vi "field emission sensor_65.vi"() -> ()   [LabVIEW 2014]
uses:
  Keithley 24XX/Public/Data/Read (Single Point).vi
  Keithley 24XX/Keithley 24XX.lvlib
  <userlib>/Nanonis Prog Interface V5/Nanonis Prog Interface.lvlib
panel:
  out "x+y":sgl
  in  "p ramp":dbl=10500.0
  out "amplitude":sgl(graph)
  in  "delay  coarse step":u32
  in  "Amplitude (V) (NaN=no change)":sgl=nan
  in  "Frequency (Hz) (NaN=no change)":sgl=nan format="%#_6p"
  in  "p Amplitude":dbl=2e-08 format="%#_6p"
  in  "amplitude max":sgl=1e-10 format="%#_6p"
  in  "Signal index (0-79)":i8=49
  out "amplitude":sgl=7.943678e-12 format="%#_6p"
  in  "dz":dbl=1e-09 format="%#_6p"
  in  "ramp delay (s)":dbl=10500.0
  out "ramp trigger":bool
  out "millisecond timer value":u32=183946603
  in  "Clear plots":bool
  out "z":dbl(graph)=1.0959994182086754e-07
  in  "Ramp":bool=TRUE
  in  "steps":sgl=5e-09 format="%#_6p"
  in  "Ramp to":sgl=2.45e-07 format="%#_6p"
  in  "I":sgl=5e-05 format="%#_6p"
  in  "PID":bool
  in  "p":sgl=0.005 format="%#_6p"
  in  "setpoint":sgl=2.5000006e-07 format="%#_3p"
  in  "max Current":sgl=1e-06 format="%#_6p"
  in  "setpoint approach":sgl=3e-08 format="%#_6p"
  in  "auto approach":bool
  in  "Number of steps":u16=1
  in  "withdraw tip":bool
  in  "coarse step":bool
  in  "Direction":enum16{"X +", "X -", "Y +", "Y -", "Z +", "Z -"}(ring)=enum."Z +"
  in  "Machine name (local machine IP)":string="localhost"
  in  "Z position [m]":dbl=1.0959994182086754e-07 max=1.096e-07 step=1.0 format="%_6p"
  out "current [A]":sgl=2.086008e-11 format="%#_6p"
  in  "time divider":dbl=60.0
  out "time elapsed":dbl=58.44645961125692
  in  "milliseconds to wait":u32=100
  in  "VISA resource name":refnum<visa-resource-name>="GPIB0::21::INSTR"
  in  "stop":bool
  in  "current multiplier":sgl=1.0
  out "Current":sgl(graph)=2.086008e-11
  # "STOP the VI during an Nanonis Auto Approach"
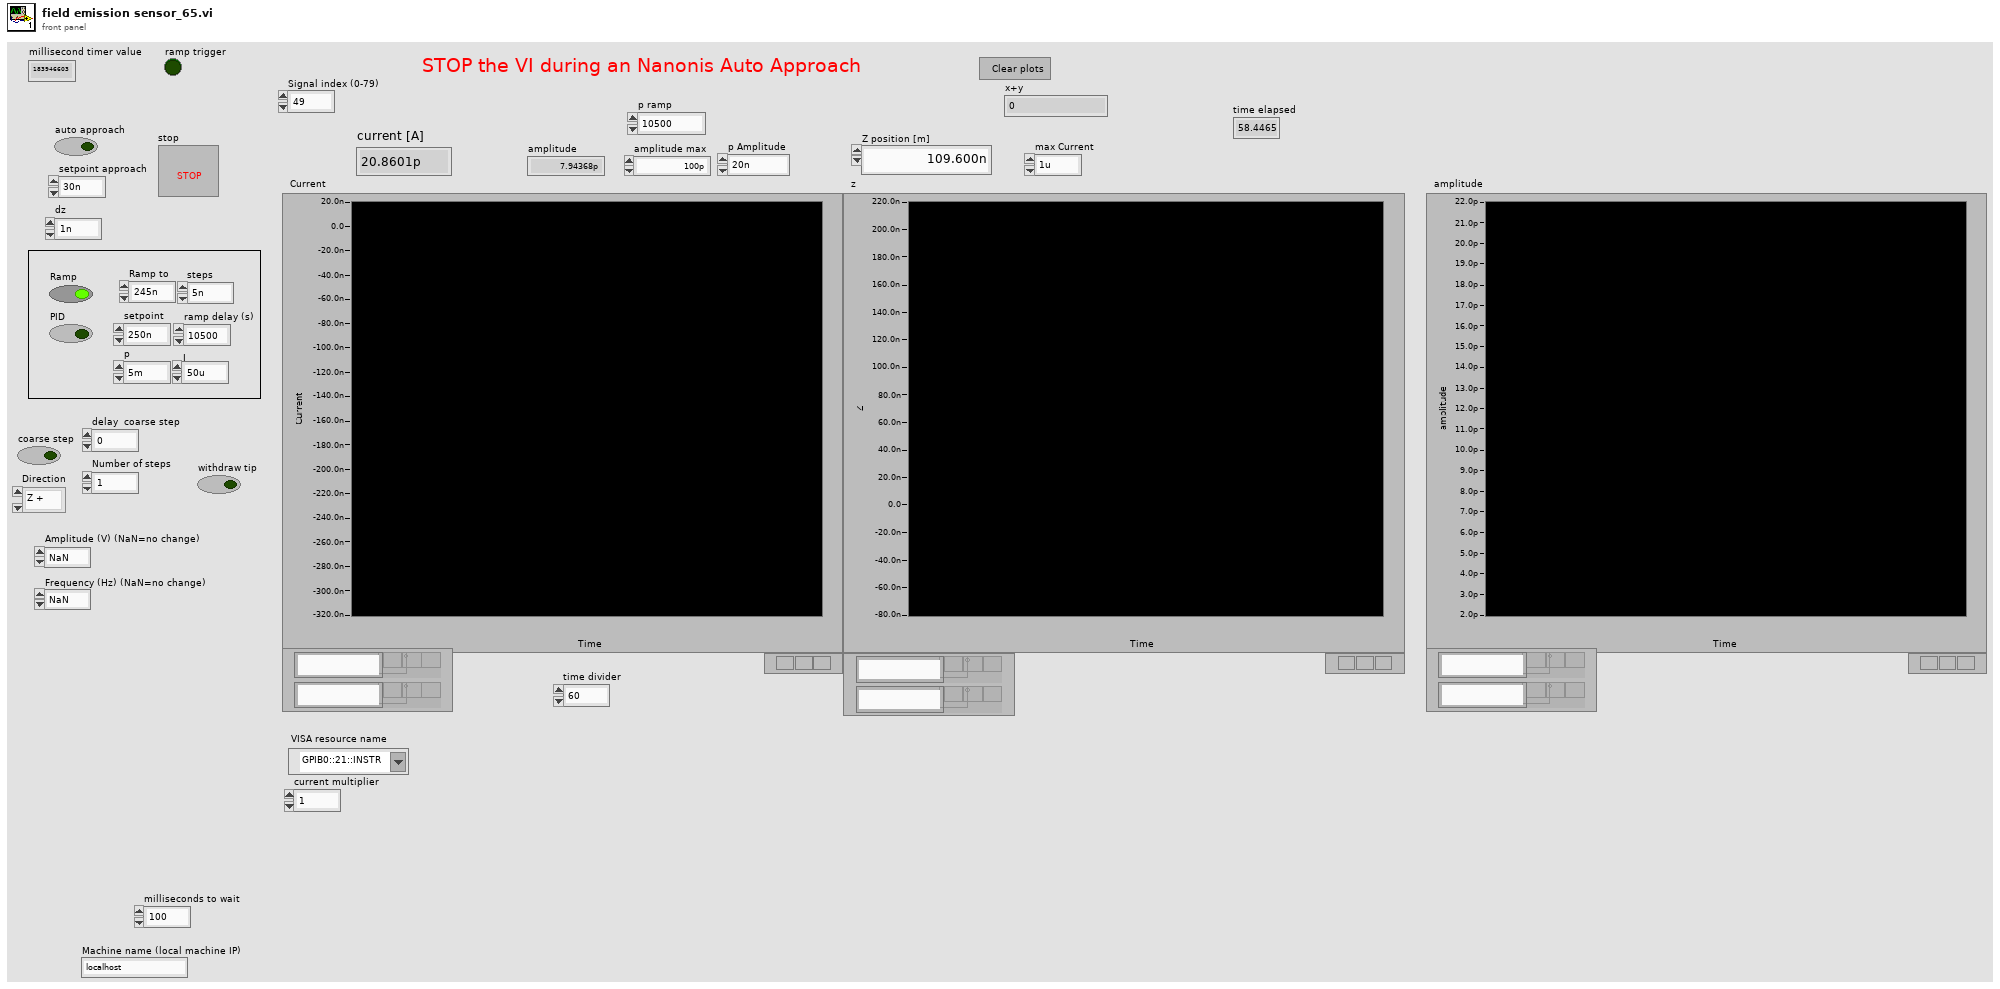
[diagram p1: front panel]
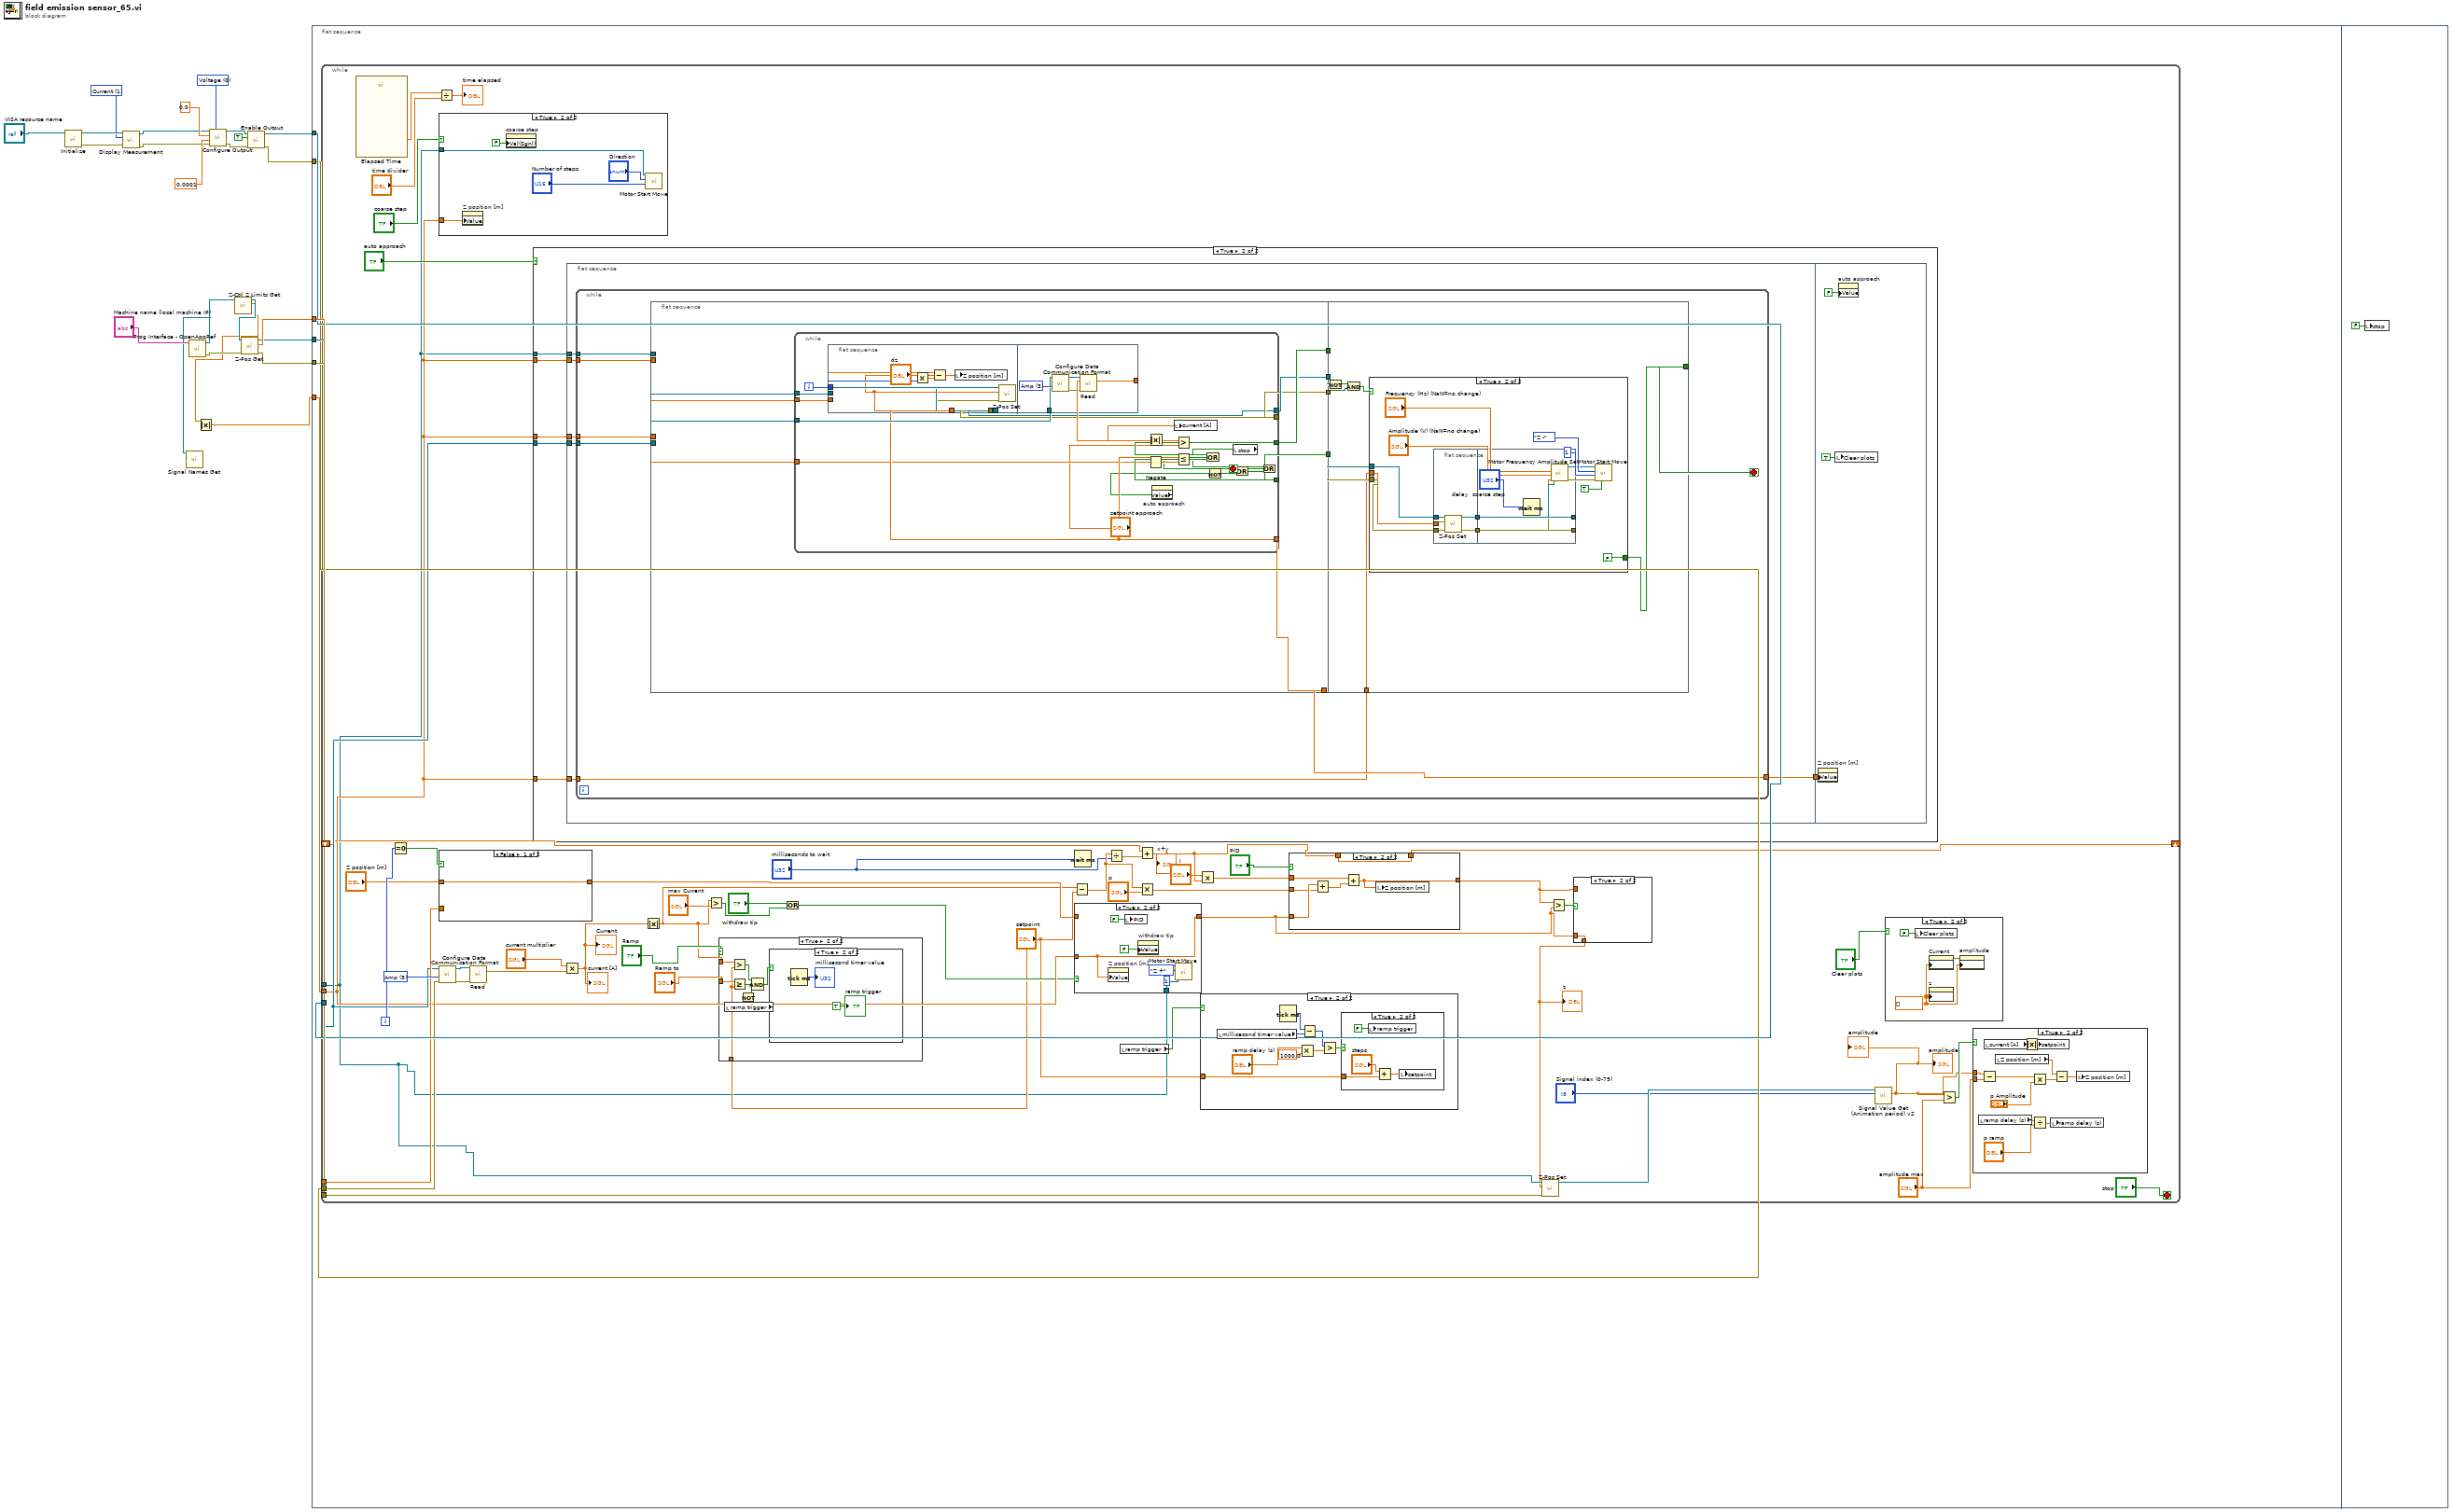
[diagram p0: block diagram]
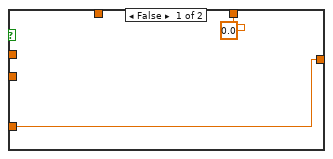
[diagram p9: hidden frame]
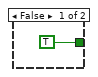
[diagram p11: hidden frame]
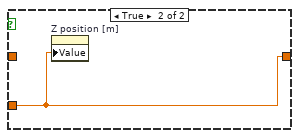
[diagram p14: hidden frame]
diagram:
  w5 = u16 1 items=["Voltage", "Current", "Resistance"] ("Displayed Measurement (0: Voltage)")
  w17 = u16 0 items=["Voltage", "Current"] ("Source Mode  (0: Voltage)")
  n1 = call "Initialize.vi"("VISA resource name"="VISA resource name") -> ("error out"=w7:errorcluster, "VISA resource name out"=w9:refnum<visa-resource-name>)  [unwired: 9 in]
  n2 = call "Display Measurement.vi"("error in (no error)"=w7, "Displayed Measurement (0: Voltage)"=w5, "VISA resource name"=w9) -> ("error out"=w6:errorcluster, "VISA resource name out"=w8:refnum<visa-resource-name>)  [unwired: 7 in]
  n3 = call <userlib>:"Prog Interface - OpenAppRef.vi"("Machine name (local machine IP)"="Machine name (local machine IP)") -> ("Error out"=w22:errorcluster, "Application reference"=w1:refnum<vi>)  [unwired: 5 in]
  n4 = call <userlib>:"Signal Names Get.vi"("Application ref in"=w1) -> ()  [unwired: 6 in, 3 out]
  n5 = call "Configure Output.vi"("Source Mode  (0: Voltage)"=w17, "error in (no error)"=w6, "Compliance  Level (0.1)"=0.0001, "Output Level (0)"=0.0, "VISA resource name"=w8) -> ("error out"=w13:errorcluster, "VISA resource name out"=w14:refnum<visa-resource-name>)  [unwired: 5 in]
  n6 = call <userlib>:"Z-Ctrl Z Limits Get.vi"("Application ref in"=w1) -> ("Z high limit"=w2:sgl, "Application ref out"=w3:refnum<vi>)  [unwired: 7 in, 2 out]
  n7 = Absolute Value(x=w2) -> (abs(x)=w4:sgl)
  n8 = call <userlib>:"Z-Pos Get.vi"("error in (no error)"=w22, "Application ref in"=w3) -> ("error out"=w21:errorcluster, "Z position (m)"=w20:sgl, "Application ref out"=w19:refnum<vi>)  [unwired: 7 in]
  n9 = call "Enable Output.vi"("error in (no error)"=w13, "Enable Output (T: Enable)"=TRUE, "VISA resource name"=w14) -> ("error out"=w10:errorcluster, "VISA resource name out"=w11:refnum<visa-resource-name>)  [unwired: 7 in]
  n10 = flat-sequence {
    tunnel: w21 -> [w29]
    tunnel: w20 -> [w28]
    tunnel: w19 -> [w27]
    tunnel: w11 -> [w26]
    tunnel: w10 -> [w25]
    tunnel: w4 -> [w24]
    frame #0 {
      n11 = while {
        tunnel: w27 -> [w34]
        tunnel: w29 -> [w73]
        tunnel: w28 -> [w72]
        tunnel: w26 -> [w64]
        tunnel: w25 -> [w63]
        tunnel: w24 -> [w61]
        shift-right: [w46] -> _
        shift-left: _ -> [w53]
        i -> [w71]
        stop <- "stop" stop-if-true
        w77 = u16 3 items=["All", "Volt and Amp", "Volt", "Amp"] ("Data Selection (0: All)")
        n12 = call "Elapsed Time"() -> ("Elapsed Time (s)"=w74:dbl)  [unwired: 12 in, 7 out]
        n13 = Equal To 0?(x=w71) -> (x = 0?=w70:bool)
        n14 = Divide(x=w74, y="time divider") -> (x/y=→"time elapsed":dbl)
        n15 = case shown="True" "coarse step" {
          tunnel: w34 -> [_ w240]
          tunnel: w61 -> [_ w236]
          frame False {
          }
          frame True {
            n16 = property on="Z position [m]" class="DigNum (strict)"("Value"=w236) -> ()  [unwired: 2 in, 2 out]
            n17 = property on="coarse step" class="Bool (strict)"("Val(Sgnl)"=FALSE ("Value (Signaling)")) -> ()  [unwired: 2 in, 2 out]
            n18 = call <userlib>:"Motor Start Move.vi"("Number of steps"="Number of steps", "Direction"="Direction", "Application ref in"=w240) -> ()  [unwired: 6 in, 2 out]
          }
        }
        n19 = case shown="False" w70 {
          tunnel: [w241 w242] -> w67
          tunnel: w72 -> [_ w242]
          tunnel: "Z position [m]" -> [w241 _]
          frame False {
          }
          frame True {
            n20 = property on="Z position [m]" class="DigNum (strict)"("Value"=w242) -> ()  [unwired: 2 in, 2 out]
          }
        }
        n21 = call "Configure Data Communication Format.vi"("error in (no error)"=w63, "Data Selection (0: All)"=w77, "VISA resource name"=w64) -> ("error out"=w78:errorcluster, "VISA resource name out"=w79:refnum<visa-resource-name>)  [unwired: 7 in]
        n22 = call-poly "Read.vi"("VISA resource name"=w79, "error in (no error)"=w78) -> ("Current"=w81:sgl)  [unwired: 7 in, 6 out]
        n23 = case shown="True" "auto approach" {
          tunnel: w64 -> [_ w134]
          tunnel: w34 -> [_ w133]
          tunnel: w61 -> [_ w131]
          tunnel: w61 -> [_ w130]
          tunnel: w61 -> [_ w129]
          frame False {
          }
          frame True {
            n24 = flat-sequence {
              tunnel: w134 -> [w140]
              tunnel: w133 -> [w139]
              tunnel: [w138] -> w132
              tunnel: w131 -> [w137]
              tunnel: w130 -> [w136]
              tunnel: w129 -> [w135]
              tunnel: w132 -> [w227]
              frame #0 {
                n25 = while {
                  tunnel: w140 -> [w151]
                  tunnel: w139 -> [w150]
                  tunnel: [w144] -> w138
                  tunnel: w137 -> [w143]
                  tunnel: w136 -> [w142]
                  tunnel: w135 -> [w141]
                  stop <- w145 stop-if-true
                  n26 = flat-sequence {
                    tunnel: w151 -> [w160]
                    tunnel: w150 -> [w159]
                    tunnel: [w158] -> w149
                    tunnel: [w157] -> w148
                    tunnel: [w156] -> w147
                    tunnel: [w155] -> w146
                    tunnel: [w154] -> w144
                    tunnel: w143 -> [w153]
                    tunnel: w141 -> [w152]
                    tunnel: w149 -> [w201]
                    tunnel: w148 -> [w199]
                    tunnel: w147 -> [w197]
                    tunnel: w146 -> [w196]
                    tunnel: [w195] -> w145
                    tunnel: w142 -> [w194]
                    frame #0 {
                      n27 = while {
                        tunnel: w160 -> [w179]
                        tunnel: w159 -> [w177]
                        tunnel: [w176] -> w158
                        tunnel: [w175] -> w157
                        tunnel: [w174] -> w156
                        tunnel: [w173] -> w155
                        tunnel: [w172] -> w154
                        tunnel: w153 -> [w171]
                        tunnel: w152 -> [w169]
                        i -> [w180]
                        stop <- w164 stop-if-true
                        n28 = flat-sequence {
                          tunnel: w180 -> [w188]
                          tunnel: w177 -> [w187]
                          tunnel: [w182] -> w172
                          tunnel: [w186] -> w174
                          tunnel: [w185] -> w173
                          tunnel: w171 -> [w184]
                          tunnel: w179 -> [w190]
                          tunnel: [w189] -> w178
                          frame #0 {
                            n29 = Multiply(x="dz", y=w188) -> (x*y=w183:dbl)
                            n30 = Subtract(x=w184, y=w183) -> (x-y=w182:dbl)
                            n31 = local write "Z position [m]"(w182) -> ()
                            n32 = call <userlib>:"Z-Pos Set.vi"("Z position (m)"=w182, "Application ref in"=w187) -> ("error out"=w185:errorcluster, "Application ref out"=w186:refnum<vi>)  [unwired: 8 in]
                          }
                          frame #1 {
                            w191 = u16 3 items=["All", "Volt and Amp", "Volt", "Amp"] ("Data Selection (0: All)")
                            n33 = call "Configure Data Communication Format.vi"("Data Selection (0: All)"=w191, "VISA resource name"=w190) -> ("error out"=w192:errorcluster, "VISA resource name out"=w193:refnum<visa-resource-name>)  [unwired: 8 in]
                            n34 = call-poly "Read.vi"("VISA resource name"=w193, "error in (no error)"=w192) -> ("Current"=w189:sgl)  [unwired: 7 in, 6 out]
                          }
                        }
                        n35 = Negate(x=w169) -> (-x=w170:sgl)
                        n36 = Absolute Value(x=w178) -> (abs(x)=w161:sgl)
                        n37 = property on="auto approach" class="Bool (strict)"() -> ("Value"=w167:bool)  [unwired: 2 in, 2 out]
                        n38 = local write "current [A]"(w161) -> ()
                        n39 = Greater?(x=w161, y="setpoint approach") -> (0:w176:bool)
                        n40 = Less Or Equal?(x=w172, y=w170) -> (x <= y?=w175:bool)
                        n41 = Or(x=w176, y=w175) -> (x .or. y?=w168:bool)
                        n42 = Not(x=w167) -> (.not. x?=w166:bool)
                        n43 = local read "stop"() -> (w163:bool)
                        n44 = Or(x=w168, y=w166) -> (x .or. y?=w165:bool)
                        n45 = Or(x=w163, y=w165) -> (x .or. y?=w164:bool)
                      }
                    }
                    frame #1 {
                      n46 = Not(x=w201) -> (.not. x?=w200:bool)
                      n47 = And(x=w200, y=w199) -> (x .and. y?=w198:bool)
                      n48 = case shown="True" w198 {
                        tunnel: w197 -> [_ w217]
                        tunnel: w196 -> [_ w216]
                        tunnel: [TRUE FALSE] -> w195
                        tunnel: w194 -> [_ w212]
                        frame False {
                        }
                        frame True {
                          n49 = flat-sequence {
                            tunnel: w217 -> [w222]
                            tunnel: w216 -> [w221]
                            tunnel: w212 -> [w220]
                            tunnel: [w219] -> w204
                            tunnel: [w218] -> w203
                            tunnel: [w224] -> w208
                            tunnel: [w225] -> w209
                            tunnel: w204 -> [w225]
                            tunnel: w203 -> [w224]
                            frame #0 {
                              n50 = call <userlib>:"Z-Pos Set.vi"("error in (no error)"=w221, "Z position (m)"=w220, "Application ref in"=w222) -> ("error out"=w218:errorcluster, "Application ref out"=w219:refnum<vi>)  [unwired: 7 in]
                            }
                            frame #1 {
                              n51 = Wait (ms)(milliseconds to wait="delay  coarse step") -> ()  [unwired: 1 out]
                            }
                          }
                          n52 = call <userlib>:"Motor Frequency Amplitude Set.vi"("Error in (no error)"=w208, "Amplitude (V) (NaN=no change)"="Amplitude (V) (NaN=no change)", "Frequency (Hz) (NaN=no change)"="Frequency (Hz) (NaN=no change)", "Application ref in"=w209) -> ("Error out"=w207:errorcluster, "Application ref out"=w210:refnum<vi>)  [unwired: 6 in]
                          n53 = call <userlib>:"Motor Start Move.vi"("Wait until finished? (F)"=TRUE, "Error in (no error)"=w207, "Number of steps"=u16 1, "Direction"=enum16{"X +", "X -", "Y +", "Y -", "Z +", "Z -"}."Z -", "Application ref in"=w210) -> ()  [unwired: 4 in, 2 out]
                        }
                      }
                    }
                  }
                }
              }
              frame #1 {
                n54 = property on="Z position [m]" class="DigNum (strict)"("Value"=w227) -> ()  [unwired: 2 in, 2 out]
                n55 = local write "Clear plots"(TRUE ("Clear plots")) -> ()
                n56 = property on="auto approach" class="Bool (strict)"("Value"=FALSE ("auto approach")) -> ()  [unwired: 2 in, 2 out]
              }
            }
          }
        }
        n57 = Multiply(x="current multiplier", y=w81) -> (x*y=w60:sgl)
        "Current" <- w60
        "current [A]" <- w60
        n58 = Absolute Value(x=w60) -> (abs(x)=w44:sgl)
        n59 = Greater?(x=w44, y="max Current") -> (0:w57:bool)
        n60 = case shown="True" "Ramp" {
          tunnel: w44 -> [_ w118]
          tunnel: "setpoint" -> [_ w115]
          tunnel: "Ramp to" -> [_ w116]
          frame False {
          }
          frame True {
            n61 = local read "ramp trigger"() -> (w112:bool)
            n62 = Greater?(x=w118, y=w115) -> (0:w117:bool)
            n63 = Greater Or Equal?(x=w116, y=w115) -> (x >= y?=w113:bool)
            n64 = Not(x=w112) -> (.not. x?=w111:bool)
            n65 = Compound Arithmetic op=AND(w117, w113, w111) -> (w114:bool)
            n66 = case shown="True" w114 {
              frame False {
              }
              frame True {
                n67 = Tick Count (ms)() -> (millisecond timer value=→"millisecond timer value":u32)
                "ramp trigger" <- TRUE ("ramp")
              }
            }
          }
        }
        n68 = Or(x="withdraw tip", y=w57) -> (x .or. y?=w58:bool)
        n69 = Subtract(x=w44, y="setpoint") -> (x-y=w49:sgl)
        n70 = Wait (ms)(milliseconds to wait="milliseconds to wait") -> ()  [unwired: 1 out]
        n71 = case shown="True" w58 {
          tunnel: [w229 w234] -> w30
          tunnel: w67 -> [w229 _]
          tunnel: w61 -> [_ w234]
          tunnel: w34 -> [_ w232]
          frame False {
          }
          frame True {
            n72 = property on="Z position [m]" class="DigNum (strict)"("Value"=w234) -> ()  [unwired: 2 in, 2 out]
            n73 = local write "PID"(FALSE ("PID")) -> ()
            n74 = property on="withdraw tip" class="Bool (strict)"("Value"=FALSE ("withdraw tip")) -> ()  [unwired: 2 in, 2 out]
            n75 = call <userlib>:"Motor Start Move.vi"("Number of steps"=u16 1, "Direction"=enum16{"X +", "X -", "Y +", "Y -", "Z +", "Z -"}."Z +", "Application ref in"=w232) -> ()  [unwired: 6 in, 2 out]
          }
        }
        n76 = Divide(x=w49, y="milliseconds to wait") -> (x/y=w50:sgl)
        n77 = local read "ramp trigger"() -> (w40:bool)
        n78 = Add(x=w53, y=w50) -> (x+y=w47:sgl)
        "x+y" <- w47
        n79 = Multiply(x=w49, y="p") -> (x*y=w54:sgl)
        n80 = Multiply(x="I", y=w47) -> (x*y=w51:sgl)
        n81 = case shown="True" w40 {
          tunnel: "setpoint" -> [_ w99]
          frame False {
          }
          frame True {
            n82 = local read "millisecond timer value"() -> (w102:u32)
            n83 = Tick Count (ms)() -> (millisecond timer value=w103:u32)
            n84 = Multiply(x="ramp delay (s)", y=1000.0) -> (x*y=w96:dbl)
            n85 = Subtract(x=w103, y=w102) -> (x-y=w101:u32)
            n86 = Greater?(x=w101, y=w96) -> (0:w100:bool)
            n87 = case shown="True" w100 {
              tunnel: w99 -> [_ w105]
              frame False {
              }
              frame True {
                n88 = local write "ramp trigger"(FALSE ("ramp")) -> ()
                n89 = Add(x="steps", y=w105) -> (x+y=w107:sgl)
                n90 = local write "setpoint"(w107) -> ()
              }
            }
          }
        }
        n91 = case shown="True" "PID" {
          tunnel: w30 -> [w122 w128]
          tunnel: [w122 w124] -> w32
          tunnel: w54 -> [_ w127]
          tunnel: w51 -> [_ w125]
          tunnel: w47 -> [_ w123]
          tunnel: [sgl 0.0 w123] -> w46
          frame False {
          }
          frame True {
            n92 = Add(x=w128, y=w127) -> (x+y=w126:dbl)
            n93 = Add(x=w125, y=w126) -> (x+y=w124:dbl)
            n94 = local write "Z position [m]"(w124) -> ()
          }
        }
        n95 = Greater?(x=w32, y=w30) -> (0:w33:bool)
        n96 = case shown="True" w33 {
          tunnel: w32 -> [w82 _]
          tunnel: [w82 w83] -> w31
          tunnel: w30 -> [_ w83]
          frame False {
          }
          frame True {
          }
        }
        "z" <- w31
        n97 = call <userlib>:"Z-Pos Set.vi"("error in (no error)"=w73, "Z position (m)"=w31, "Application ref in"=w34) -> ("Application ref out"=w39:refnum<vi>)  [unwired: 7 in, 1 out]
        n98 = call <userlib>:"Signal Value Get (Animation period) v2.vi"("Signal index (0-79)"="Signal index (0-79)", "Application ref in"=w39) -> ("Signal value"=w36:sgl)  [unwired: 6 in, 2 out]
        "amplitude" <- w36
        "amplitude" <- w36
        n99 = case shown="True" "Clear plots" {
          frame False {
          }
          frame True {
            w108 = dbl[] [] ("History Data")
            n100 = local write "Clear plots"(FALSE ("Clear plots")) -> ()
            n101 = property on="Current" class="WFChart (strict)"("History Data"=w108) -> (error out=w109:errorcluster)  [unwired: 2 in, 1 out]
            n102 = property on="z" class="WFChart (strict)"("History Data"=w108) -> ()  [unwired: 2 in, 2 out]
            n103 = property on="amplitude" class="WFChart (strict)"(error in=w109, "History Data"=w108) -> ()  [unwired: 1 in, 2 out]
          }
        }
        n104 = Greater?(x=w36, y="amplitude max") -> (0:w37:bool)
        n105 = case shown="True" w37 {
          tunnel: w36 -> [_ w93]
          tunnel: "amplitude max" -> [_ w92]
          frame False {
          }
          frame True {
            n106 = local read "ramp delay (s)"() -> (w87:dbl)
            n107 = Subtract(x=w93, y=w92) -> (x-y=w91:sgl)
            n108 = local read "current [A]"() -> (w88:sgl)
            n109 = local read "Z position [m]"() -> (w95:dbl)
            n110 = Absolute Value(x=w88) -> (abs(x)=w84:sgl)
            n111 = Multiply(x=w91, y="p Amplitude") -> (x*y=w89:dbl)
            n112 = Divide(x=w87, y="p ramp") -> (x/y=w85:dbl)
            n113 = local write "setpoint"(w84) -> ()
            n114 = local write "ramp delay (s)"(w85) -> ()
            n115 = Subtract(x=w95, y=w89) -> (x-y=w94:dbl)
            n116 = local write "Z position [m]"(w94) -> ()
          }
        }
      }
    }
    frame #1 {
      n117 = local write "stop"(FALSE ("stop")) -> ()
    }
  }
